vi "select cluster.vi"(8 "error in (no error)":errorcluster, 11 "Item Ref in":T3 format="%.0x") -> (0 "error out":errorcluster, 3 "Parent Ref out":T3 format="%.0x")   [LabVIEW 2009, in "NI-XNET Custom Device.lvlib"]
uses:
  NI-XNET Custom Device.lvlib
  <vilib>/NI VeriStand/Custom Device API/Custom Device Item Ref.ctl
  <vilib>/NI VeriStand/Custom Device API/Set Item Property (String).vi
  <vilib>/xnet/xnet.llb/XNET String To IO Name (Interface).vi
  <vilib>/NI VeriStand/Custom Device API/Set Item Property (Variant).vi
  <vilib>/NI VeriStand/Custom Device API/Custom Device API.lvlib
panel:
  in  "Interface (FlexRay)":T1(ring)
  in  "Interface Type":u16(ring) items=["CAN", "FlexRay"]
  in  "Interface (CAN)":T2(ring)
  in  "OK Button":bool
  in  "Select Cluster":u16(ring) items=["nixnet_example.CAN_Cluster", "nixnet_example.CAN_Demo_Box_Cluster"]
  in  "XNET Database":refnum<k21>="nixnet_example"
  # "Custom Device"
  # "Select which type of interface you are using."
  # "Select which interface is tied to this custom device.  You cannot use the same interface for two custom devices. \n\nTo see which interfaces are available in the system, please use measurement and automation explorer."
  # "Select you XNET Database you want to associate to this custom device.  You will need to delete the custom device if you want to use another database.  Once you select a database, it is recommended that you not change the Cluster, Frame and Signal names, as this may break the custom device settings."
  # "To Browse for a database on your host machine or to edit a database, click on the control and scroll to the bottom."
  # "Select which database cluster you want to use.  For CAN, the cluster defines the baudrate of the transmission."
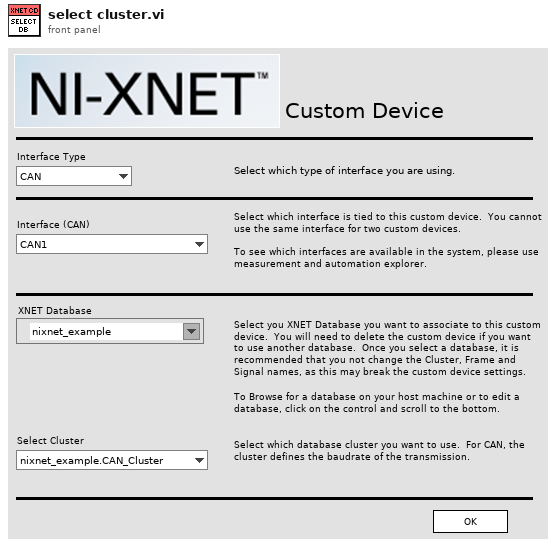
[diagram p1: front panel]
types:
  T1 = enum16{"FlexRay1", "FlexRay2", "FlexRay3", "FlexRay4", "FlexRay5", "FlexRay6", "FlexRay7", "FlexRay8", "FlexRay9", "FlexRay10", "FlexRay11", "FlexRay12", "FlexRay13", "FlexRay14", "FlexRay15", "FlexRay16", "FlexRay17", "FlexRay18", "FlexRay19", "FlexRay20"}
  T2 = enum16{"CAN1", "CAN2", "CAN3", "CAN4", "CAN5", "CAN6", "CAN7", "CAN8", "CAN9", "CAN10", "CAN11", "CAN12", "CAN13", "CAN14", "CAN15", "CAN16", "CAN17", "CAN18", "CAN19", "CAN20"}
  T3 = typedef "Custom Device API.lvlib/Custom Device Item Ref.ctl" = u64
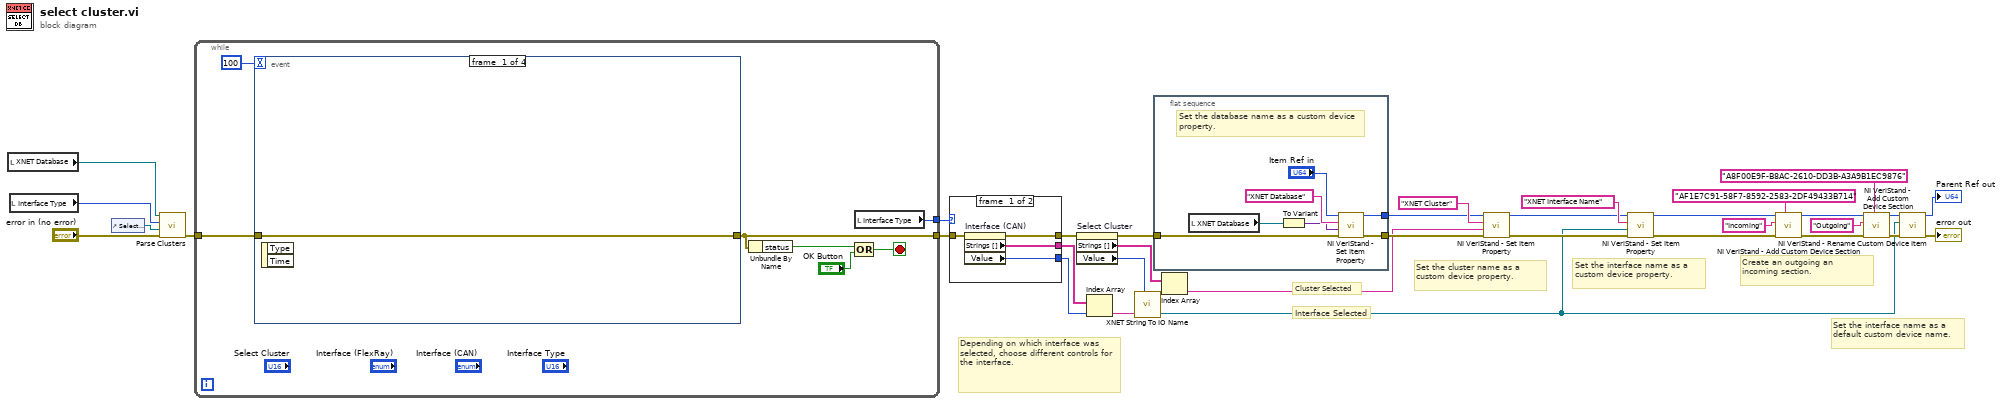
[diagram p0: block diagram]
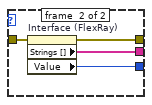
[diagram p2: hidden frame]
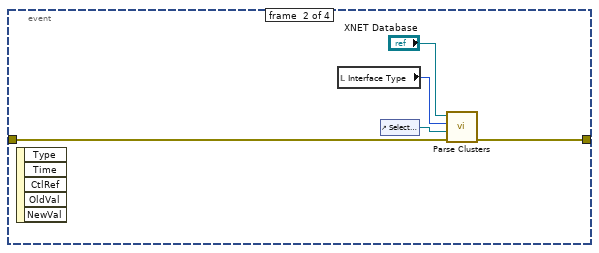
[diagram p3: hidden frame]
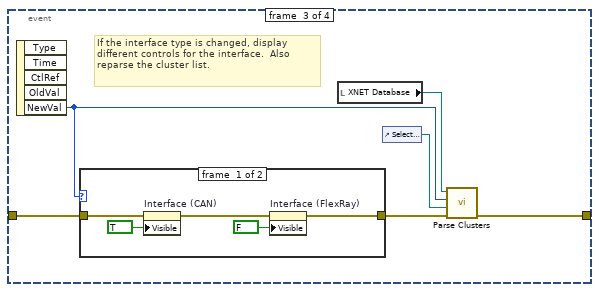
[diagram p4: hidden frame]
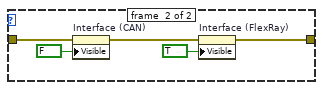
[diagram p5: hidden frame]
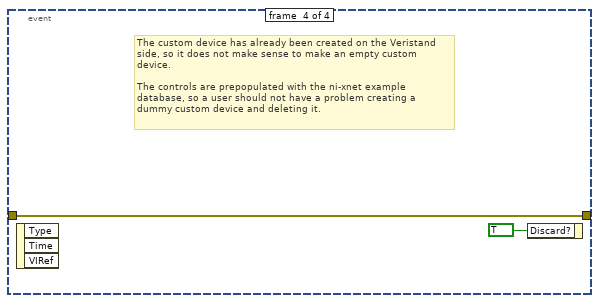
[diagram p6: hidden frame]
diagram:
  # "Create an outgoing an incoming section."
  # "Set the interface name as a default custom device name."
  # "Set the interface name as a custom device property."
  # "Set the cluster name as a custom device property."
  # "Cluster Selected"
  # "Interface Selected"
  # "Depending on which interface was selected, choose different controls for the interface."
  n1 = local read "XNET Database"() -> (w5:refnum<k21>)
  n2 = local read "Interface Type"() -> (w6:u16)
  n3 = control-ref of="Select Cluster"() -> (w4:refnum<vi>)
  n4 = call "Parse Clusters.vi"("error in (no error)"="error in (no error)", "CLuster Ring"=w4, "Interface Type"=w6, "XNET Database"=w5) -> ("error out"=w7:errorcluster)  [unwired: 7 in]
  n5 = while {
    tunnel: w7 -> [w41]
    tunnel: [w39] -> w3
    tunnel: [w35] -> w2
    stop <- w38 stop-if-true
    n6 = event shown="[3] Panel Close?" {
      selector: _ -> [_ _ _ _]
      dyn-events: _ -> [_ _ _ _]
      timeout: 100 -> [_ _ _ _]
      tunnel: w41 -> [w42 w46 w53 w64]
      tunnel: [w42 w47 w51 w64] -> w39
      event #0 {
        n7 = event-data() -> ()  [unwired: 1 in, 2 out]
      }
      event #1 {
        n8 = event-data() -> ()  [unwired: 1 in, 5 out]
        n9 = local read "Interface Type"() -> (w43:u16)
        n10 = control-ref of="Select Cluster"() -> (w45:refnum<vi>)
        n11 = call "Parse Clusters.vi"("error in (no error)"=w46, "CLuster Ring"=w45, "Interface Type"=w43, "XNET Database"="XNET Database") -> ("error out"=w47:errorcluster)  [unwired: 7 in]
      }
      event #2 {
        # "If the interface type is changed, display different controls for the interface.  Also reparse the cluster list."
        n12 = event-data() -> ("NewVal"=w49:u16)  [unwired: 1 in, 4 out]
        n13 = case shown="1" w49 {
          tunnel: w53 -> [w55 w61]
          tunnel: [w54 w59] -> w52
          frame #0 {
            n14 = property on="Interface (CAN)" class="Enum (strict)"(error in=w55, "Visible"=TRUE) -> (error out=w56:errorcluster)  [unwired: 1 in, 1 out]
            n15 = property on="Interface (FlexRay)" class="Enum (strict)"(error in=w56, "Visible"=FALSE) -> (error out=w54:errorcluster)  [unwired: 1 in, 1 out]
          }
          frame #1 {
            n16 = property on="Interface (CAN)" class="Enum (strict)"(error in=w61, "Visible"=FALSE) -> (error out=w60:errorcluster)  [unwired: 1 in, 1 out]
            n17 = property on="Interface (FlexRay)" class="Enum (strict)"(error in=w60, "Visible"=TRUE) -> (error out=w59:errorcluster)  [unwired: 1 in, 1 out]
          }
        }
        n18 = local read "XNET Database"() -> (w50:refnum<k21>)
        n19 = control-ref of="Select Cluster"() -> (w48:refnum<vi>)
        n20 = call "Parse Clusters.vi"("error in (no error)"=w52, "CLuster Ring"=w48, "Interface Type"=w49, "XNET Database"=w50) -> ("error out"=w51:errorcluster)  [unwired: 7 in]
      }
      event #3 {
        # "The custom device has already been created on the Veristand side, so it does not make sense to make an empty custom device.\n\nThe controls are prepopulated with the ni-xnet example database, so a user should not have a problem creating a dummy custom device and deleting it."
        n21 = event-data() -> ()  [unwired: 1 in, 3 out]
        n22 = event-data("Discard?"=TRUE) -> ()  [unwired: 1 in, 1 out]
      }
    }
    n23 = Unbundle By Name(w39) -> ("status"=w36:bool)
    n24 = local read "Interface Type"() -> (w35:u16)
    n25 = Compound Arithmetic op=OR(w36, "OK Button") -> (w38:bool)
  }
  n26 = case shown="1" w2 {
    tunnel: [w69 w70] -> w12
    tunnel: [w68 w71] -> w11
    tunnel: [w67 w72] -> w10
    tunnel: w3 -> [w66 w73]
    frame #0 {
      n27 = property on="Interface (CAN)" class="Enum (strict)"(error in=w66) -> (error out=w67:errorcluster, "Strings []"=w68:string[], "Value"=w69:T2)  [unwired: 1 in, 1 out]
    }
    frame #1 {
      n28 = property on="Interface (FlexRay)" class="Enum (strict)"(error in=w73) -> (error out=w72:errorcluster, "Strings []"=w71:string[], "Value"=w70:T1)  [unwired: 1 in, 1 out]
    }
  }
  n29 = property on="Select Cluster" class="Ring (strict)"(error in=w10) -> (error out=w9:errorcluster, "Strings []"=w17:string[], "Value"=w18:u16)  [unwired: 1 in, 1 out]
  n30 = Index Array(array=w11, index=w12) -> (element=w13:string)
  n31 = call-poly <vilib>:"XNET String To IO Name.vi"("string"=w13) -> ("XNET Interface"=w1:refnum<k21>)  [unwired: 4 in]
  n32 = flat-sequence {
    tunnel: [w78] -> w22
    tunnel: [w77] -> w19
    tunnel: w9 -> [w75]
    frame #0 {
      # "Set the database name as a custom device property."
      n33 = local read "XNET Database"() -> (w74:refnum<k21>)
      n34 = To Variant(anything=w74) -> (Variant=w76:variant)
      n35 = call-poly <vilib>:"NI VeriStand - Set Item Property.vi"("error in (no error)"=w75, "Value"=w76, "Property Name"="XNET Database", "Item Ref in"="Item Ref in") -> ("error out"=w78:errorcluster, "Item Ref out"=w77:T3)  [unwired: 5 in, 1 out]
    }
  }
  n36 = Index Array(array=w17, index=w18) -> (element=w14:string)
  n37 = call-poly <vilib>:"NI VeriStand - Set Item Property.vi"("error in (no error)"=w22, "Value"=w14, "Property Name"="XNET Cluster", "Item Ref in"=w19) -> ("error out"=w21:errorcluster, "Item Ref out"=w31:T3)  [unwired: 5 in, 1 out]
  n38 = call-poly <vilib>:"NI VeriStand - Set Item Property.vi"("error in (no error)"=w21, "Value"=w1, "Property Name"="XNET Interface Name", "Item Ref in"=w31) -> ("error out"=w20:errorcluster, "Item Ref out"=w30:T3)  [unwired: 5 in, 1 out]
  n39 = call <vilib>:"NI VeriStand - Add Custom Device Section.vi"("GUID (Default Section)"="AF1E7C91-58F7-8592-2583-2DF49433B714", "error in (no error)"=w20, "Section Name"="Incoming", "Parent Ref in"=w30) -> ("error out"=w25:errorcluster, "Parent Ref out"=w24:T3)  [unwired: 5 in, 1 out]
  n40 = call <vilib>:"NI VeriStand - Add Custom Device Section.vi"("GUID (Default Section)"="A8F00E9F-B8AC-2610-DD3B-A3A9B1EC9876", "error in (no error)"=w25, "Section Name"="Outgoing", "Parent Ref in"=w24) -> ("error out"=w16:errorcluster, "Parent Ref out"=w15:T3)  [unwired: 5 in, 1 out]
  n41 = call <vilib>:"NI VeriStand - Rename Custom Device Item.vi"("error in (no error)"=w16, "New Name"=w1, "Item Ref in"=w15) -> ("error out"=→"error out":errorcluster, "Item Ref out"=→"Parent Ref out":T3)  [unwired: 6 in, 1 out]
